vi "Write System Log Ref.vi"(8 "error in (no error)":errorcluster, 10 "System Log":refnum<vi>, 11 "Log Indicator in":refnum<class "Log Indicator.lvclass">) -> (0 "error out":errorcluster, 3 "Log Indicator out":refnum<class "Log Indicator.lvclass">)   [LabVIEW 2020, in "Log Indicator.lvclass"]
uses:
  Log Indicator.lvclass
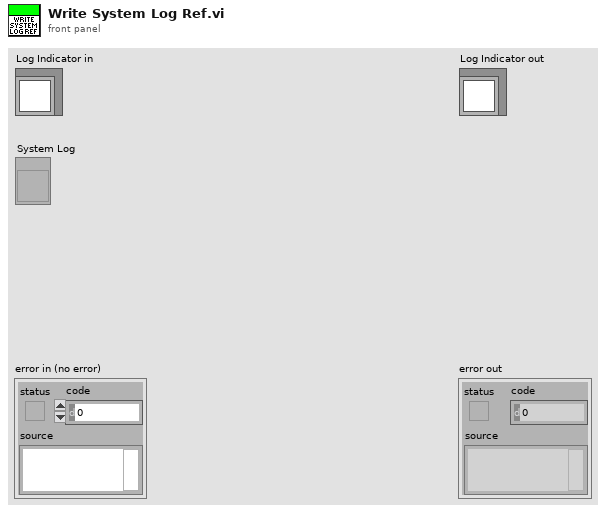
[diagram p1: front panel]
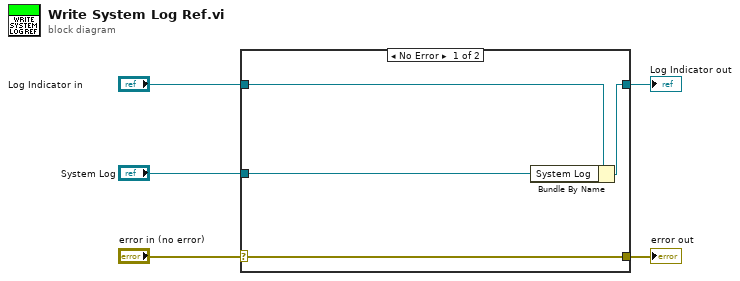
[diagram p0: block diagram]
diagram:
  n1 = case shown="No Error" "error in (no error)" {
    selector: "error in (no error)" -> [w9 w10]
    tunnel: [w9 w10] -> w4
    tunnel: [w7 w11] -> w2
    tunnel: "Log Indicator in" -> [w8 w11]
    tunnel: "System Log" -> [w6 _]
    frame No Error {
      n2 = Bundle By Name(cluster=w8, "System Log"=w6) -> (w7:refnum<class "Log Indicator.lvclass">)
    }
    frame Error {
    }
  }
  "error out" <- w4
  "Log Indicator out" <- w2
